vi "Manually Test Script.vi"(5 "Copy Script Into Window":string="generate HV29", 8 "Error In":errorcluster, 11 "HSDIO Sessions":T1) -> (0 "Error Out":errorcluster)   [LabVIEW 2013]
uses:
  <instrlib>/niHSDIO/niHSDIO.llb/niHSDIO_ctl Generation Mode Values (Ring).ctl
  <instrlib>/niHSDIO/niHSDIO.llb/niHSDIO_ctl Trigger Script - trigID Values (Ring).ctl
  <instrlib>/niHSDIO/niHSDIO.llb/niHSDIO_ctl Trigger SW - TrigName Values (Ring).ctl
  <instrlib>/niHSDIO/niHSDIO.llb/niHSDIO_ctl Trigger SW - TrigIdentifier Values (Ring).ctl
  <instrlib>/niHSDIO/niHSDIO.llb/niHSDIO Configure Software Script Trigger.vi
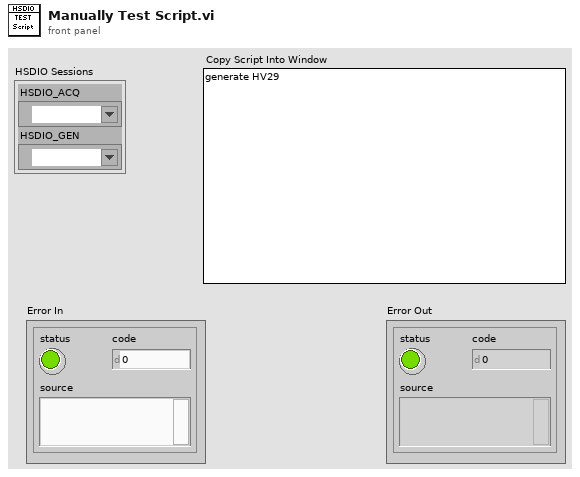
[diagram p1: front panel]
types:
  T1 = cluster{"HSDIO_ACQ":refnum<k15>, "HSDIO_GEN":refnum<k15>}
  T2 = typedef "niHSDIO_ctl Trigger Script - trigID Values (Ring).ctl" = string
  T3 = typedef "niHSDIO_ctl Generation Mode Values (Ring).ctl" = i32
  T4 = typedef "niHSDIO_ctl Trigger SW - TrigIdentifier Values (Ring).ctl" = string
  T5 = typedef "niHSDIO_ctl Trigger SW - TrigName Values (Ring).ctl" = i32
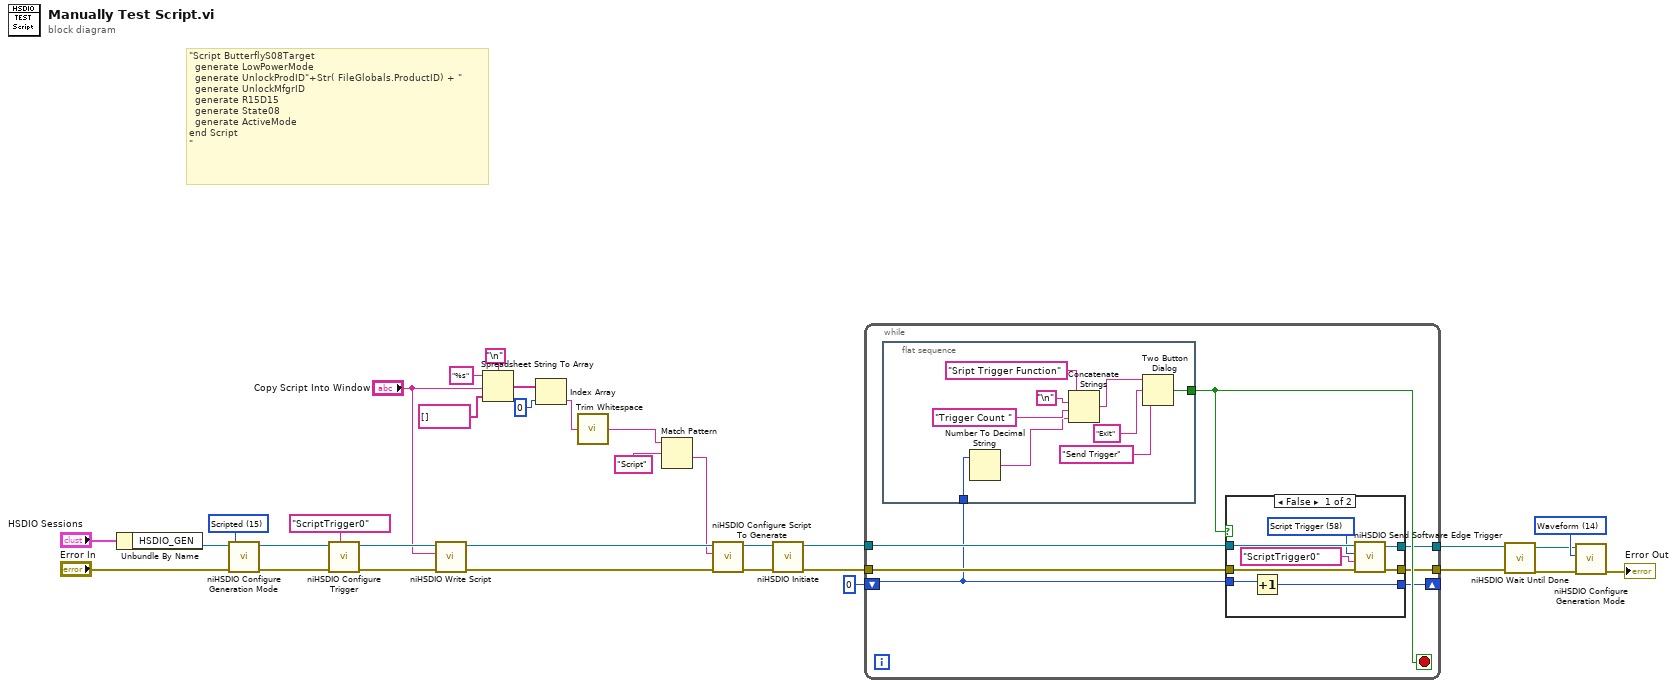
[diagram p0: block diagram]
diagram:
  w29 = T3 14 items=["Waveform"=14, "Scripted"=15] ("generation mode (waveform)")
  w30 = T3 15 items=["Waveform"=14, "Scripted"=15] ("generation mode (waveform)")
  # "\"Script ButterflyS08Target\n  generate LowPowerMode\n  generate UnlockProdID\"+Str( FileGlobals.ProductID) + \"\n  generate UnlockMfgrID\n  generate R15D15\n  generate State08\n  generate ActiveMode\nend Script\n\""
  n1 = Unbundle By Name("HSDIO Sessions") -> ("HSDIO_GEN"=w23:refnum<k15>)
  n2 = call <instrlib>:"niHSDIO Configure Generation Mode.vi"("error in (no error)"="Error In", "generation mode (waveform)"=w30, "instrument handle"=w23) -> ("error out"=w18:errorcluster, "instrument handle out"=w19:refnum<k15>)  [unwired: 7 in]
  n3 = call-poly <instrlib>:"niHSDIO Configure Trigger.vi"("trigger id (script trigger 0)"=T2 "ScriptTrigger0", "error in (no error)"=w18, "instrument handle"=w19) -> ("error out"=w17:errorcluster, "instrument handle out"=w16:refnum<k15>)  [unwired: 7 in]
  n4 = call <instrlib>:"niHSDIO Write Script.vi"("error in (no error)"=w17, "script"="Copy Script Into Window", "instrument handle"=w16) -> ("error out"=w32:errorcluster, "instrument handle out"=w31:refnum<k15>)  [unwired: 7 in]
  n5 = Spreadsheet String To Array(delimiter (Tab)="\n", format string="%s", spreadsheet string="Copy Script Into Window", array type (2D Dbl)=string[] []) -> (array=w12:string[])
  n6 = Index Array(array=w12, index=0) -> (element=w9:string)
  n7 = call <vilib>:"Trim Whitespace.vi"("string"=w9) -> ("trimmed string"=w2:string)  [unwired: 1 in]
  n8 = Match Pattern(string=w2, regular expression="Script") -> (after substring=w7:string)  [unwired: 1 in, 3 out]
  n9 = call <instrlib>:"niHSDIO Configure Script To Generate.vi"("error in (no error)"=w32, "script name"=w7, "instrument handle"=w31) -> ("error out"=w27:errorcluster, "instrument handle out"=w28:refnum<k15>)  [unwired: 7 in]
  n10 = call <instrlib>:"niHSDIO Initiate.vi"("error in (no error)"=w27, "instrument handle"=w28) -> ("error out"=w6:errorcluster, "instrument handle out"=w5:refnum<k15>)  [unwired: 8 in]
  n11 = while {
    tunnel: w6 -> [w38]
    tunnel: [w37] -> w4
    tunnel: w5 -> [w36]
    tunnel: [w35] -> w3
    shift-right: [w34] -> _
    shift-left: 0 -> [w33]
    stop <- w39 stop-if-true
    n12 = flat-sequence {
      tunnel: [w57] -> w39
      tunnel: w33 -> [w53]
      frame #0 {
        n13 = Number To Decimal String(number=w53) -> (decimal integer string=w51:string)  [unwired: 1 in]
        n14 = Concatenate Strings("Sript Trigger Function" ("message"), "\n", "Trigger Count " ("message"), w51) -> (w56:string)
        n15 = Two Button Dialog(message=w56, 1:"Send Trigger" ("T button name (\"OK\")"), 2:"Exit" ("F button name (\"Cancel\")")) -> (T button?=w57:bool)
      }
    }
    n16 = case shown="False" w39 {
      tunnel: w38 -> [w47 w50]
      tunnel: [w46 w50] -> w37
      tunnel: w36 -> [w45 w49]
      tunnel: [w44 w49] -> w35
      tunnel: w33 -> [w41 w48]
      tunnel: [w40 w48] -> w34
      frame False {
        w43 = T5 58 items=["Start Trigger"=53, "Reference Trigger"=54, "Advance Trigger"=61, "Script Trigger"=58, "Stop Trigger"=82] ("trigger (start trigger)")
        n17 = Increment(x=w41) -> (x+1=w40:i32)
        n18 = call <instrlib>:"niHSDIO Send Software Edge Trigger.vi"("error in (no error)"=w47, "trigger identifier (none)"=T4 "ScriptTrigger0", "trigger (start trigger)"=w43, "instrument handle"=w45) -> ("error out"=w46:errorcluster, "instrument handle out"=w44:refnum<k15>)  [unwired: 6 in]
      }
      frame True {
      }
    }
  }
  n19 = call <instrlib>:"niHSDIO Wait Until Done.vi"("error in (no error)"=w4, "instrument handle"=w3) -> ("error out"=w26:errorcluster, "instrument handle out"=w25:refnum<k15>)  [unwired: 8 in]
  n20 = call <instrlib>:"niHSDIO Configure Generation Mode.vi"("error in (no error)"=w26, "generation mode (waveform)"=w29, "instrument handle"=w25) -> ("error out"=→"Error Out":errorcluster)  [unwired: 7 in, 1 out]
